vi "XMLIsCurrentFileVersion.vi"(0 "Path":string, 5 "TS.InputStream in":refnum<k7>, 9 "Index":i32) -> (4 "IsCurrentFileVersion":i32, 14 "ErrorMsg out":string, 15 "ErrorEnum out":i32)   [LabVIEW 2011]
uses:
  HelperVIsforXMLTranslator.llb/XMLarrayglobal.vi
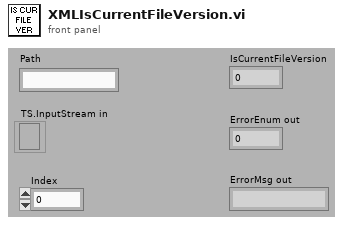
[diagram p1: front panel]
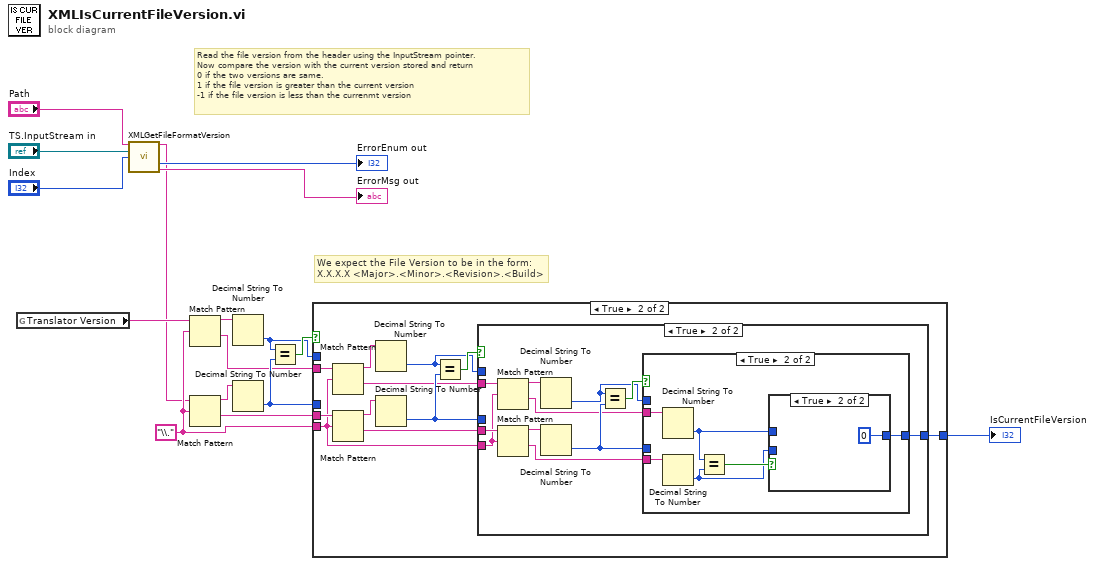
[diagram p0: block diagram]
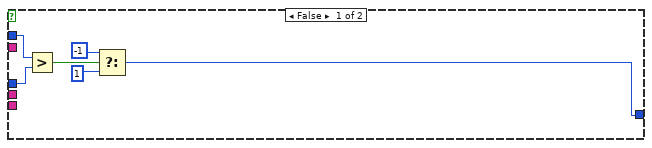
[diagram p2: hidden frame]
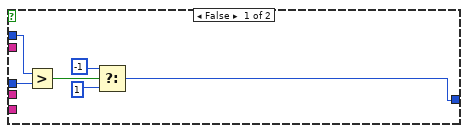
[diagram p3: hidden frame]
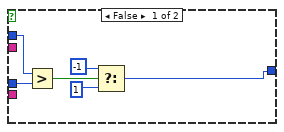
[diagram p4: hidden frame]
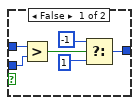
[diagram p5: hidden frame]
diagram:
  w9 = "\\." ("regular expression")
  # "We expect the File Version to be in the form:\nX.X.X.X <Major>.<Minor>.<Revision>.<Build>"
  # "Read the file version from the header using the InputStream pointer.\nNow compare the version with the current version stored and return\n0 if the two versions are same.\n1 if the file version is greater than the current version\n-1 if the file version is less than the currenmt version"
  n1 = global read "XMLarrayglobal.vi" "Translator Version"() -> (w8:string)
  n2 = call "XMLGetFileFormatVersion.vi"("Path"="Path", "TS.InputStream in"="TS.InputStream in", "Index"="Index") -> ("FileFormatVersion out"=w1:string, "ErrorEnum out"=→"ErrorEnum out":i32, "ErrMsg out"=→"ErrorMsg out":string)  [unwired: 10 in]
  n3 = Match Pattern(string=w8, regular expression=w9) -> (before substring=w16:string, after substring=w11:string)  [unwired: 1 in, 2 out]
  n4 = Match Pattern(string=w1, regular expression=w9) -> (before substring=w15:string, after substring=w10:string)  [unwired: 1 in, 2 out]
  n5 = Decimal String To Number(string=w16) -> (number=w13:i32)  [unwired: 2 in, 1 out]
  n6 = Decimal String To Number(string=w15) -> (number=w12:i32)  [unwired: 2 in, 1 out]
  n7 = Equal?(x=w13, y=w12) -> (x = y?=w14:bool)
  n8 = case shown="True" w14 {
    tunnel: w11 -> [_ w27]
    tunnel: w10 -> [_ w26]
    tunnel: w13 -> [w22 _]
    tunnel: w12 -> [w21 _]
    tunnel: [w17 w28] -> w7
    tunnel: w9 -> [_ w23]
    frame False {
      n9 = Greater?(x=w22, y=w21) -> (0:w20:bool)
      n10 = Select(t=-1, s=w20, f=1 ("t")) -> (s? t:f=w17:i32)
    }
    frame True {
      n11 = Match Pattern(string=w27, regular expression=w23) -> (before substring=w33:string, after substring=w24:string)  [unwired: 1 in, 2 out]
      n12 = Match Pattern(string=w26, regular expression=w23) -> (before substring=w32:string, after substring=w25:string)  [unwired: 1 in, 2 out]
      n13 = Decimal String To Number(string=w33) -> (number=w30:i32)  [unwired: 2 in, 1 out]
      n14 = Decimal String To Number(string=w32) -> (number=w29:i32)  [unwired: 2 in, 1 out]
      n15 = Equal?(x=w30, y=w29) -> (x = y?=w31:bool)
      n16 = case shown="True" w31 {
        tunnel: w24 -> [_ w44]
        tunnel: w30 -> [w36 _]
        tunnel: w29 -> [w35 _]
        tunnel: w25 -> [_ w43]
        tunnel: [w34 w45] -> w28
        tunnel: w23 -> [_ w40]
        frame False {
          n17 = Greater?(x=w36, y=w35) -> (0:w39:bool)
          n18 = Select(t=-1, s=w39, f=1 ("t")) -> (s? t:f=w34:i32)
        }
        frame True {
          n19 = Match Pattern(string=w44, regular expression=w40) -> (before substring=w50:string, after substring=w41:string)  [unwired: 1 in, 2 out]
          n20 = Match Pattern(string=w43, regular expression=w40) -> (before substring=w49:string, after substring=w42:string)  [unwired: 1 in, 2 out]
          n21 = Decimal String To Number(string=w50) -> (number=w47:i32)  [unwired: 2 in, 1 out]
          n22 = Decimal String To Number(string=w49) -> (number=w46:i32)  [unwired: 2 in, 1 out]
          n23 = Equal?(x=w47, y=w46) -> (x = y?=w48:bool)
          n24 = case shown="True" w48 {
            tunnel: w47 -> [w53 _]
            tunnel: w46 -> [w52 _]
            tunnel: [w51 w59] -> w45
            tunnel: w42 -> [_ w57]
            tunnel: w41 -> [_ w58]
            frame False {
              n25 = Greater?(x=w53, y=w52) -> (0:w56:bool)
              n26 = Select(t=-1, s=w56, f=1 ("t")) -> (s? t:f=w51:i32)
            }
            frame True {
              n27 = Decimal String To Number(string=w58) -> (number=w61:i32)  [unwired: 2 in, 1 out]
              n28 = Decimal String To Number(string=w57) -> (number=w60:i32)  [unwired: 2 in, 1 out]
              n29 = Equal?(x=w61, y=w60) -> (x = y?=w62:bool)
              n30 = case shown="True" w62 {
                tunnel: w61 -> [w65 _]
                tunnel: w60 -> [w64 _]
                tunnel: [w63 0 ("t")] -> w59
                frame False {
                  n31 = Greater?(x=w65, y=w64) -> (0:w68:bool)
                  n32 = Select(t=-1, s=w68, f=1 ("t")) -> (s? t:f=w63:i32)
                }
                frame True {
                }
              }
            }
          }
        }
      }
    }
  }
  "IsCurrentFileVersion" <- w7
